vi "Finish.vi"(8 "Error In":errorcluster, 11 "Lexer In":refnum<class "Lexer.lvclass">) -> (0 "Error Out":errorcluster, 3 "Lexer Out":refnum<class "Lexer.lvclass">)   [LabVIEW 2018, in "Toolkit.lvlib" / "Lexer.lvclass"]
uses:
  Lexer.lvclass
  Lexer.lvclass/Lexer.ctl
  Tokens/Text/Text.lvclass
  D:/Users/cfield/Code/Field R&D Services/Labstache/src/Toolkit/Low-Level/Tokens/Token/Token.lvclass
  Tokens/EscapedVariable/EscapedVariable.lvclass
  Tokens/Comment/Comment.lvclass
  Tokens/UnescapedVariable/UnescapedVariable.lvclass
  Tokens/BeginSection/BeginSection.lvclass
  Tokens/InvertedSection/InvertedSection.lvclass
  Tokens/EndSection/EndSection.lvclass
  Tokens/Partial/Partial.lvclass
  Tokens/Text/New.vi
  <vilib>/Utility/error.llb/Trim Whitespace.vi
  Tokens/EscapedVariable/New.vi
  Tokens/Comment/New.vi
  Tokens/UnescapedVariable/New.vi
  Tokens/BeginSection/New.vi
  Tokens/InvertedSection/New.vi
  Tokens/EndSection/New.vi
  Tokens/Partial/New.vi
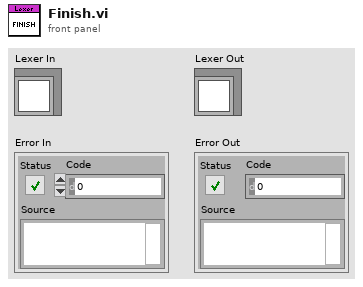
[diagram p1: front panel]
types:
  T1 = typedef "Toolkit.lvlib/Lexer.lvclass/States.ctl" = enum16{"Text", "Open Delimiter", "Tag Type", "Tag Key", "Close Delimiter"}
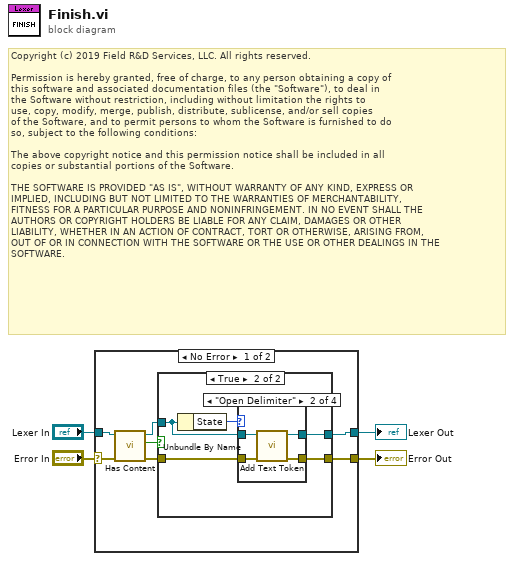
[diagram p0: block diagram]
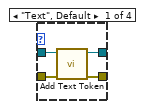
[diagram p3: hidden frame]
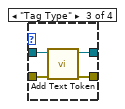
[diagram p4: hidden frame]
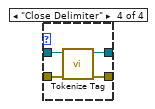
[diagram p5: hidden frame]
diagram:
  # "Copyright (c) 2019 Field R&D Services, LLC. All rights reserved.\n\nPermission is hereby granted, free of charge, to any person obtaining a copy of\nthis software and associated documentation files (the \"Software\"), to deal in\nthe Software without restriction, including without limitation the rights to\nuse, copy, modify, merge, publish, distribute, sublicense, and/or sell copies\nof the Software, and to permit persons to whom the Software is furnished to do\nso, subject to the following conditions:\n\nThe above copyright notice and this permission notice shall be included in all\ncopies or substantial portions of the Software.\n\nTHE SOFTWARE IS PROVIDED \"AS IS\", WITHOUT WARRANTY OF ANY KIND, EXPRESS OR\nIMPLIED, INCLUDING BUT NOT LIMITED TO THE WARRANTIES OF MERCHANTABILITY,\nFITNESS FOR A PARTICULAR PURPOSE AND NONINFRINGEMENT. IN NO EVENT SHALL THE\nAUTHORS OR COPYRIGHT HOLDERS BE LIABLE FOR ANY CLAIM, DAMAGES OR OTHER\nLIABILITY, WHETHER IN AN ACTION OF CONTRACT, TORT OR OTHERWISE, ARISING FROM,\nOUT OF OR IN CONNECTION WITH THE SOFTWARE OR THE USE OR OTHER DEALINGS IN THE\nSOFTWARE."
  n1 = case shown="No Error" "Error In" {
    selector: "Error In" -> [w5 w35]
    tunnel: [w11 w36] -> w4
    tunnel: "Lexer In" -> [w7 w36]
    tunnel: [w6 w35] -> w2
    frame No Error {
      n2 = call "Has Content.vi"("Error In"=w5, "Lexer In"=w7) -> ("Error Out"=w10:errorcluster, "Content"=w8:bool, "Lexer Out"=w9:refnum<class "Lexer.lvclass">)  [unwired: 7 in]
      n3 = case shown="True" w8 {
        tunnel: w9 -> [w12 w17]
        tunnel: w10 -> [w13 w16]
        tunnel: [w12 w15] -> w11
        tunnel: [w13 w14] -> w6
        frame False {
        }
        frame True {
          n4 = Unbundle By Name(w17) -> ("State"=w18:T1)
          n5 = case shown="\"Open Delimiter\"" w18 {
            tunnel: w17 -> [w22 w26 w30 w34]
            tunnel: w16 -> [w21 w23 w27 w31]
            tunnel: [w20 w24 w28 w32] -> w14
            tunnel: [w19 w25 w29 w33] -> w15
            frame "Text", Default {
              n6 = call "Add Text Token.vi"("Error In"=w21, "Lexer In"=w22) -> ("Error Out"=w20:errorcluster, "Lexer Out"=w19:refnum<class "Lexer.lvclass">)  [unwired: 8 in]
            }
            frame "Open Delimiter" {
              n7 = call "Add Text Token.vi"("Error In"=w23, "Lexer In"=w26) -> ("Error Out"=w24:errorcluster, "Lexer Out"=w25:refnum<class "Lexer.lvclass">)  [unwired: 8 in]
            }
            frame "Tag Type" {
              n8 = call "Add Text Token.vi"("Error In"=w27, "Lexer In"=w30) -> ("Error Out"=w28:errorcluster, "Lexer Out"=w29:refnum<class "Lexer.lvclass">)  [unwired: 8 in]
            }
            frame "Close Delimiter" {
              n9 = call "Tokenize Tag.vi"("Error In"=w31, "Lexer In"=w34) -> ("Error Out"=w32:errorcluster, "Lexer Out"=w33:refnum<class "Lexer.lvclass">)  [unwired: 8 in]
            }
          }
        }
      }
    }
    frame Error {
    }
  }
  "Lexer Out" <- w4
  "Error Out" <- w2
